vi "Initialize Identity Attribute.vi"(9 "Prospective Owner":string, 10 "Unique Name":string, 11 "Given Name":string) -> (2 "GUID":string, 3 "Attribute.Identity":refnum<class "Attribute.Identity.lvclass">)   [LabVIEW 2021, in "smo.lvlib" / "Attribute.Identity.lvclass"]
uses:
  Attribute.Identity.lvclass
  C:/Repositories/SMO/src/Support/Attribute/Attribute.lvclass
  Definitions/def.SMO/Scope -- Enum.ctl
  Attribute/Attribute.lvclass/Attribute.ctl
  Attribute.Identity.lvclass/Attribute.Identity.ctl
  Definitions/def.SMO/def.SMO.lvclass
  Attribute/Attribute.lvclass
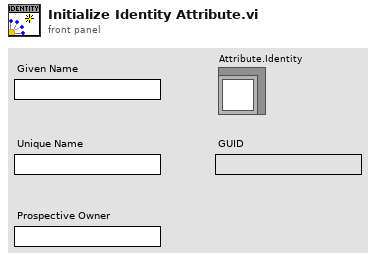
[diagram p1: front panel]
types:
  T1 = typedef "smo.lvlib/def.SMO.lvclass/Scope -- Enum.ctl" = enum16{"Public", "Protected", "Private"}
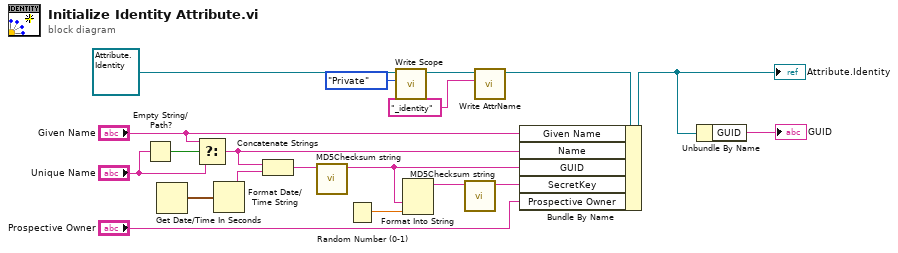
[diagram p0: block diagram]
diagram:
  n1 = Empty String/Path?(string/path="Unique Name") -> (empty?=w10:bool)
  n2 = Get Date/Time In Seconds() -> (seconds since 1Jan1904=w19:timestamp)
  n3 = Select(t="Given Name", s=w10, f="Unique Name") -> (s? t:f=w7:string)
  n4 = Format Date/Time String(seconds (now)=w19) -> (date/time string=w18:string)  [unwired: 2 in]
  n5 = Concatenate Strings(w7, w18) -> (w17:string)
  n6 = call <vilib>:"MD5Checksum string.vi"("Message String"=w17) -> ("MD5 message-digest"=w13:string)  [unwired: 10 in]
  n7 = Random Number (0-1)() -> (number: 0 to 1=w16:dbl)
  n8 = call "Write Scope.vi"("Scope"=Scope_--_Enum."Private", "Attribute in"=refnum<class "Attribute.Identity.lvclass"> refnum ("Attribute.Owner in")) -> ("Attribute out"=w3:refnum<class "Attribute.Identity.lvclass">)  [unwired: 9 in]
  n9 = Format Into String(w13, w16) -> (resulting string=w15:string)  [unwired: 3 in, 1 out]
  n10 = call <vilib>:"MD5Checksum string.vi"("Message String"=w15) -> ("MD5 message-digest"=w14:string)  [unwired: 10 in]
  n11 = call "Write AttrName.vi"("Attribute Name"="_identity", "Attribute in"=w3) -> ("Attribute out"=w1:refnum<class "Attribute.Identity.lvclass">)  [unwired: 9 in]
  n12 = Bundle By Name(cluster=w1, "Given Name"="Given Name", "Name"=w7, "GUID"=w13, "SecretKey"=w14, "Prospective Owner"="Prospective Owner") -> (w12:refnum<class "Attribute.Identity.lvclass">)
  "Attribute.Identity" <- w12
  n13 = Unbundle By Name(w12) -> ("GUID"=→"GUID":string)
